vi "fill_elements_by_name_from_target.vi"(5 "little-endian arrays (T)":bool=TRUE, 8 "error in (no error)":errorcluster, 10 "arrayOfElements":T1[](array[typedef]), 11 "dataType in":variant) -> (0 "error out":errorcluster, 3 "dataType out":variant)   [LabVIEW 2015, in "BSON_convertors_Library.lvlib"]
uses:
  BSON_convertors_Library.lvlib
  typedefs/BSONelement.ctl
  typedefs/dataType.ctl
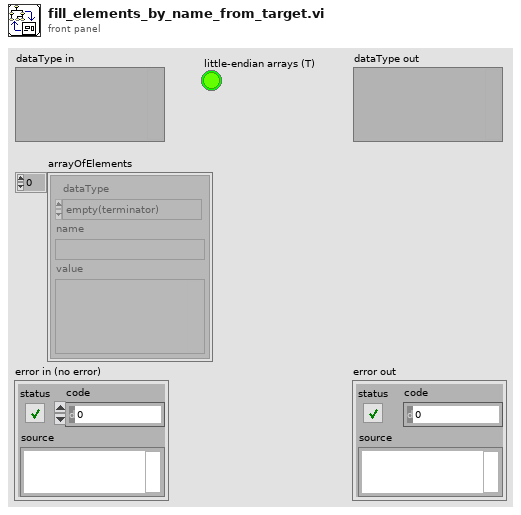
[diagram p1: front panel]
types:
  T1 = typedef "BSON_convertors_Library.lvlib/BSONelement.ctl" = cluster{"dataType":T2, "name":string, "value":variant}
  T2 = typedef "BSON_convertors_Library.lvlib/dataType.ctl" = enum8{"empty(terminator)", "double", "string", "document", "array", "binary", "Deprecated(Undefined)", "ObjectId", "boolean", "UTC datetime", "Null value", "cstring", "Deprecated(DBPointer)", "JavaScript", "Deprecated(Symbol)", "code_w_s", "int32", "uint64", "int64", "ext (decimal128)", "Min key", "Max key"}
  T3 = typedef "Type Descriptor Enumeration__ogtk.ctl" = enum8{"<Null>", "I8", "I16", "I32", "I64", "U8", "U16", "U32", "U64", "SGL", "DBL", "EXT", "CSG", "CDB", "CXT", "0x0F", "0x10", "0x11", "0x12", "0x13", "0x14", "Enum U8", "Enum U16", "Enum U32", "Enum U64", "SGL PQ", "DBL PQ", "EXT PQ", "CSG PQ", "CDB PQ", "CXT PQ", "0x1F", "0x20", "Boolean", "0x22", "0x23", "0x24", "0x25", "0x26", "0x27", "0x28", "0x29", "0x2A", "0x2B", "0x2C", "0x2D", "0x2E", "0x2F", "String", "0x31", "Path", "Pict", "0x34", "0x35", "0x36", "DAQ", "0x38", "0x39", "0x3A", "0x3B", "0x3C", "0x3D", "0x3E", "0x3F", "Array", "0x41", "0x42", "0x43", "0x44", "0x45", "0x46", "0x47", "0x48", "0x49", "0x4A", "0x4B", "0x4C", "0x4D", "0x4E", "0x4F", "Cluster", "0x51", "0x52", "Variant", "Waveform", "0x55", "0x56", "0x57", "0x58", "0x59", "0x5A", "0x5B", "0x5C", "0x5D", "0x5E", "0x5F", "0x60", "0x61", "0x62", "0x63", "0x64", "0x65", "0x66", "0x67", "0x68", "0x69", "0x6A", "0x6B", "0x6C", "0x6D", "0x6E", "0x6F", "Refnum"}
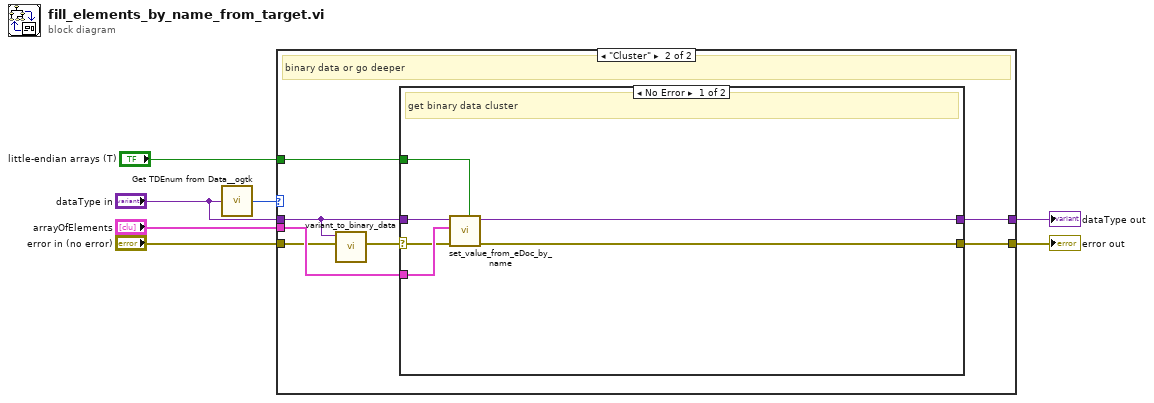
[diagram p0: block diagram]
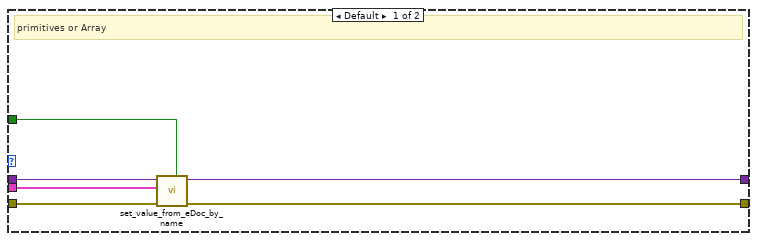
[diagram p2: hidden frame]
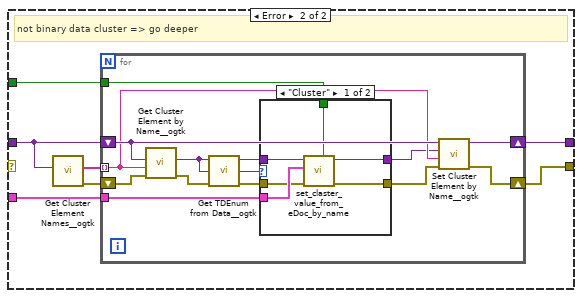
[diagram p3: hidden frame]
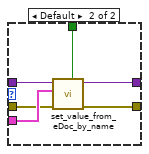
[diagram p4: hidden frame]
diagram:
  n1 = call <userlib>:"Get TDEnum from Data__ogtk.vi"("Data"="dataType in") -> ("Type Descriptor Enumeration"=w7:T3)  [unwired: 4 in]
  n2 = case shown="\"Cluster\"" w7 {
    tunnel: "arrayOfElements" -> [w12 w20]
    tunnel: "dataType in" -> [w13 w16]
    tunnel: [w11 w19] -> w4
    tunnel: "error in (no error)" -> [w9 w15]
    tunnel: [w10 w18] -> w2
    tunnel: "little-endian arrays (T)" -> [w8 w17]
    frame Default {
      # "primitives or Array"
      n3 = call "set_value_from_eDoc_by_name.vi"("little-endian?"=w8, "error in (no error)"=w9, "arrayOfElements"=w12, "dataType in"=w13) -> ("error out"=w10:errorcluster, "Data dup"=w11:variant)  [unwired: 6 in]
    }
    frame "Cluster" {
      # "binary data or go deeper"
      n4 = call "variant_to_binary_data.vi"("error in (no error)"=w15, "DataIn"=w16) -> ("error out"=w14:errorcluster)  [unwired: 8 in, 1 out]
      n5 = case shown="No Error" w14 {
        selector: w14 -> [w24 _]
        tunnel: w20 -> [w25 w32]
        tunnel: [w23 w30] -> w19
        tunnel: [w22 w29] -> w18
        tunnel: w17 -> [w21 w28]
        tunnel: w16 -> [w26 w27]
        frame No Error {
          # "get binary data cluster"
          n6 = call "set_value_from_eDoc_by_name.vi"("little-endian?"=w21, "error in (no error)"=w24, "arrayOfElements"=w25, "dataType in"=w26) -> ("error out"=w22:errorcluster, "Data dup"=w23:variant)  [unwired: 6 in]
        }
        frame Error {
          # "not binary data cluster => go deeper"
          n7 = call <userlib>:"Get Cluster Element Names__ogtk.vi"("Cluster"=w27) -> ("error out"=w31:errorcluster, "Element Names"=w33:string[])  [unwired: 9 in]
          n8 = for {
            tunnel: w33 -> [w43] mode=indexing
            tunnel: w32 -> [w40]
            shift-right: [w36] -> w29
            shift-left: w31 -> [w45]
            shift-right: [w42] -> w30
            shift-left: w27 -> [w44]
            tunnel: w28 -> [w34]
            n9 = call <userlib>:"Get Cluster Element by Name__ogtk.vi"("error in (no error)"=w45, "Element Name"=w43, "Cluster"=w44) -> ("error out"=w39:errorcluster, "VElement"=w41:variant)  [unwired: 6 in, 1 out]
            n10 = call <userlib>:"Get TDEnum from Data__ogtk.vi"("Data"=w41) -> ("Type Descriptor Enumeration"=w35:T3)  [unwired: 4 in]
            n11 = case shown="\"Cluster\"" w35 {
              tunnel: w41 -> [w51 w57]
              tunnel: w40 -> [w49 w56]
              tunnel: w39 -> [w48 w55]
              tunnel: [w50 w54] -> w38
              tunnel: [w47 w53] -> w37
              tunnel: w34 -> [w46 w52]
              frame "Cluster" {
                n12 = call "set_claster_value_from_eDoc_by_name.vi"("little-endian arrays (T)"=w46, "error in (no error)"=w48, "arrayOfElements"=w49, "dataType in"=w51) -> ("error out"=w47:errorcluster, "Data dup"=w50:variant)  [unwired: 6 in]
              }
              frame Default {
                n13 = call "set_value_from_eDoc_by_name.vi"("little-endian?"=w52, "error in (no error)"=w55, "arrayOfElements"=w56, "dataType in"=w57) -> ("error out"=w53:errorcluster, "Data dup"=w54:variant)  [unwired: 6 in]
              }
            }
            n14 = call <userlib>:"Set Cluster Element by Name__ogtk.vi"("error in (no error)"=w37, "Element Name (\"\": New Element Data Name)"=w43, "New Element Value"=w38, "Cluster"=w44) -> ("error out"=w36:errorcluster, "VCluster out"=w42:variant)  [unwired: 5 in, 1 out]
          }
        }
      }
    }
  }
  "dataType out" <- w4
  "error out" <- w2
